vi "SP_DEMO.vi"() -> ()   [LabVIEW 2009]
panel:
  out "ASM":string
  # "This LabVIEW item is deprecated.\n\nIt is believed to be unused and will be removed in a future version of SRV."
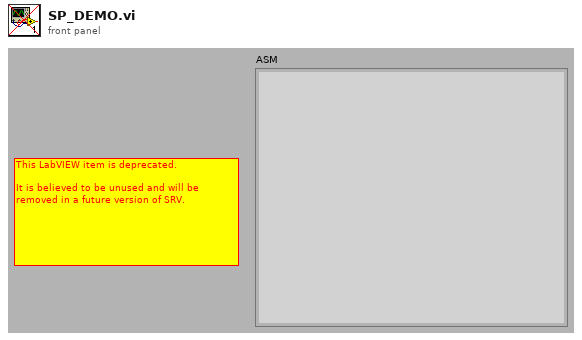
[diagram p1: front panel]
types:
  T1 = typedef "SuperProControl.ctl" = cluster{"Task":i32, "Indent":i32, "Err":i32, "ASM":string}
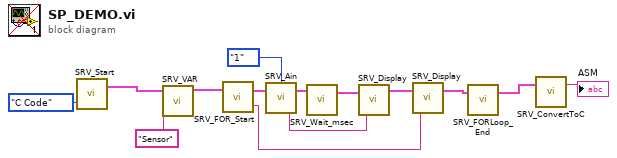
[diagram p0: block diagram]
diagram:
  n1 = call "SRV_Start.vi"("Target"=enum16{"PC", "SRV", "C Code"}."C Code") -> ("SuperPro"=w4:T1)  [unwired: 3 in]
  n2 = call "SRV_VAR.vi"("SuperPro in"=w4, "Name"="Sensor") -> ("SuperPro out"=w3:T1)  [unwired: 1 in, 3 out]
  n3 = call "SRV_FOR_Start.vi"("SuperPro"=w3) -> ("Counter"=w5:string, "SuperPro"=w14:T1)  [unwired: 2 in]
  n4 = call "SRV_Ain.vi"("SuperPro"=w14, "Channel"=enum16{"1", "2", "3", "4", "5"}."1") -> ("Variable Out"=w6:string, "SuperPro"=w13:T1)  [unwired: 1 in]
  n5 = call "SRV_Wait_msec.vi"("SuperPro"=w13) -> ("SuperPro"=w10:T1)  [unwired: 3 in]
  n6 = call "SRV_Display.vi"("Variable Name"=w6, "SuperPro"=w10) -> ("SuperPro"=w8:T1)  [unwired: 2 in]
  n7 = call "SRV_Display.vi"("Variable Name"=w5, "SuperPro"=w8) -> ("SuperPro"=w7:T1)  [unwired: 2 in]
  n8 = call "SRV_FORLoop_End.vi"("SuperPro"=w7) -> ("SuperPro"=w12:T1)  [unwired: 3 in]
  n9 = call "SRV_ConvertToC.vi"("SuperPro"=w12) -> ("C"=→"ASM":string)  [unwired: 1 in, 1 out]
